vi "GetGtagKeyValue.vi"(1 "tag":string, 2 "parameters":cluster{"key":string, "value":string}[](array[cluster])) -> (0 "value":string)   [LabVIEW 2012]
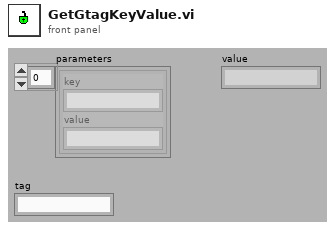
[diagram p1: front panel]
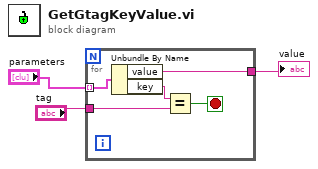
[diagram p0: block diagram]
diagram:
  n1 = for {
    tunnel: "parameters" -> [w8] mode=indexing
    tunnel: "tag" -> [w6]
    tunnel: [w4] -> w3
    stop <- w5 stop-if-true
    n2 = Unbundle By Name(w8) -> ("value"=w4:string, "key"=w7:string)
    n3 = Equal?(x=w7, y=w6) -> (x = y?=w5:bool)
  }
  "value" <- w3
